vi "PLC to MES monitor - old.vi"(0 "UTP IO Session in":T1, 5 "Sequence Context In":refnum<k7>, 7 "Logged In":bool, 9 "Packaging Performed":bool, 11 "error in":errorcluster) -> (4 "UTP IO Session out":T1, 15 "error out":errorcluster)   [LabVIEW 2023]
uses:
  <vilib>/Noffz/UTP IO/UTP IO Library/Typedefs/Session Handle.ctl
  <vilib>/Noffz/UTP IO/UTP IO Library/UTP IO Pool Session.lvclass
  MES/RequestData.ctl
  5ea416fa-7da9-46cf-b64f-edb3a1b9c4c5.vi
  <vilib>/Noffz/UTP IO/UTP IO Library/methods/poly/plc/Read PLC Variable (Boolean).vi
  <vilib>/Noffz/UTP IO/UTP IO Library/methods/poly/plc/Write PLC Variable (Boolean).vi
  <vilib>/Noffz/UTP IO/UTP IO Library/methods/poly/plc/Write PLC Variable (I16).vi
  <vilib>/addons/TestStand/_TSUtility.llb/TestStand - Get Property Value (Boolean).vi
  <vilib>/addons/TestStand/_TSUtility.llb/TestStand - Get Property Value (String).vi
panel:
  in  "stop":bool
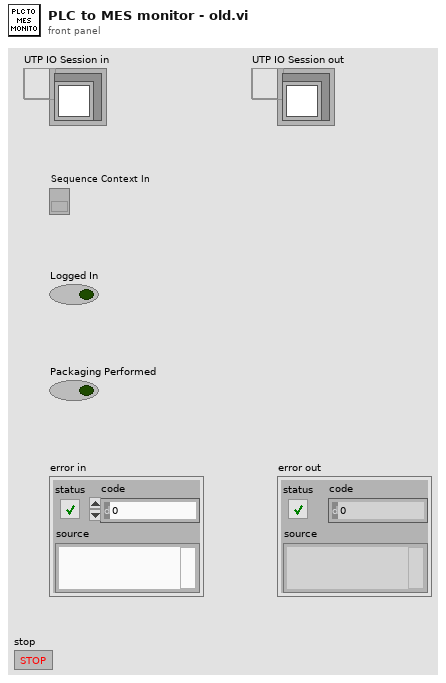
[diagram p1: front panel]
types:
  T1 = typedef "UTP IO Library.lvlib/UTP IO Pool Session.lvclass/Session Handle.ctl" = refnum<data-value>
  T2 = typedef "RequestData.ctl" = cluster{"SOAP":cluster{"HuNo":string, "MaterialCode":string, "Mode":i32, "Operator":string, "PackingInstructions":string, "ProductionVersion":string, "SerialNo":string}, "HU Validation":cluster{"MaterialCode":string, "Operator":string, "SerialNo":string}, "Login":cluster{"EquipmentCode":string, "Mode":i32, "Operator":string}}
  T3 = typedef "TestStand - Status Monitor.ctl" = cluster{"Sequence Context":refnum<k7>, "Execution":refnum<k7>, "Termination Monitor":refnum<k7>}
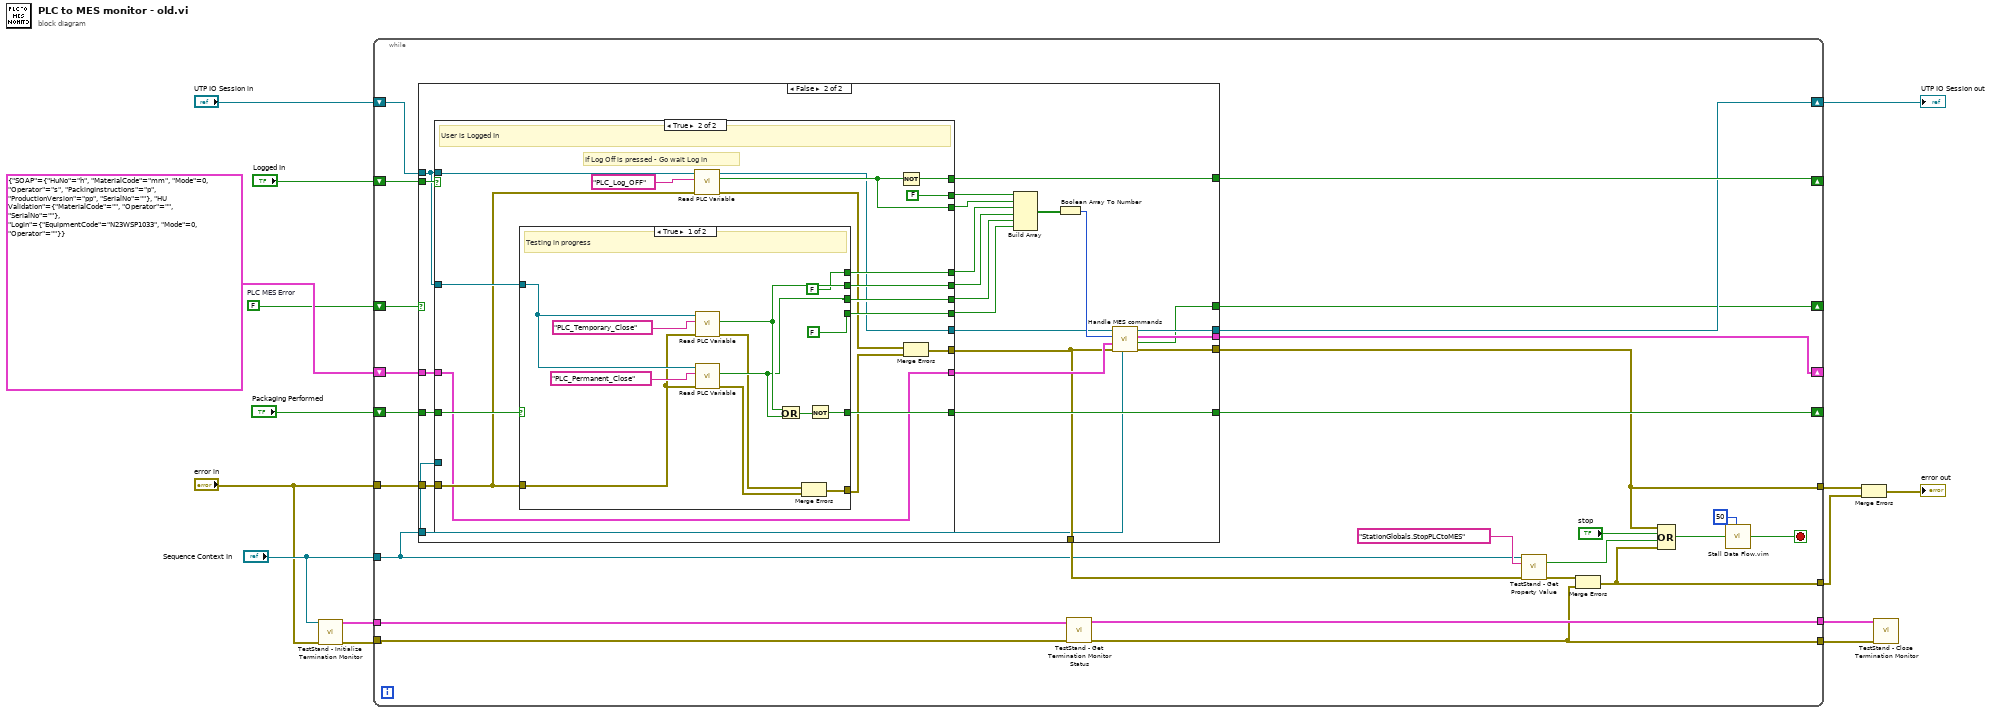
[diagram p0: block diagram]
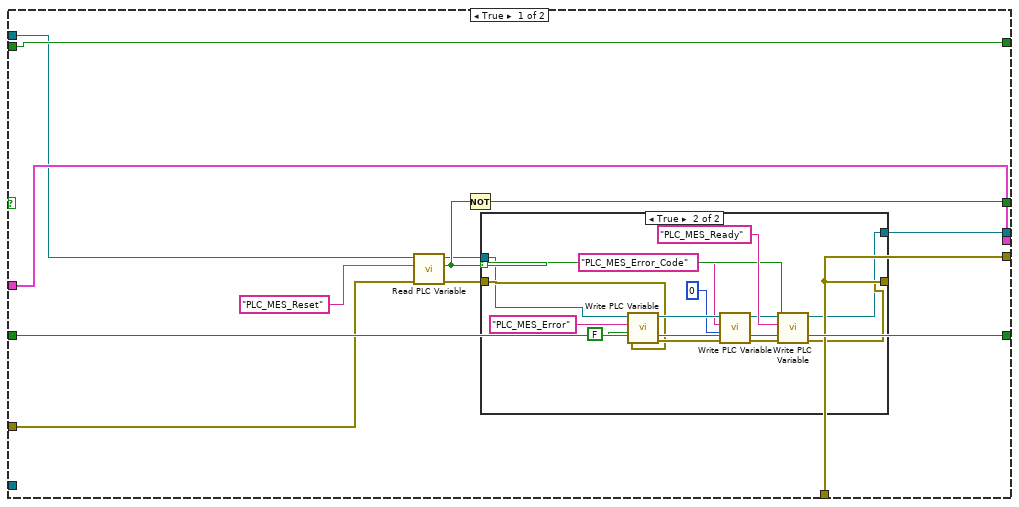
[diagram p2: hidden frame]
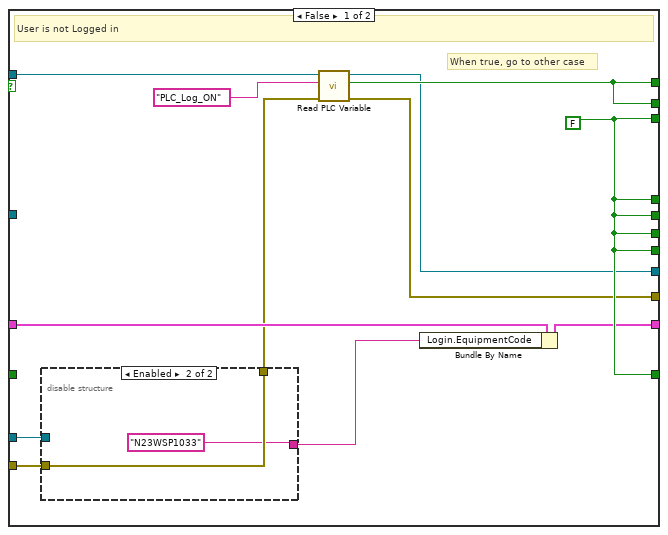
[diagram p4: hidden frame]
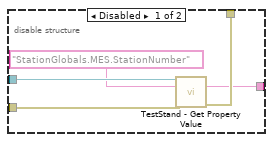
[diagram p5: hidden frame]
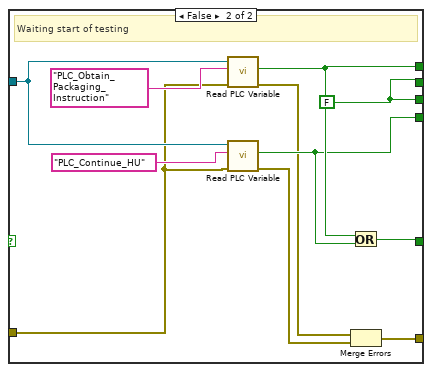
[diagram p6: hidden frame]
diagram:
  w1 = FALSE  # PLC MES Error
  n1 = call <vilib>:"TestStand - Initialize Termination Monitor.vi"("error in (no error)"="error in", "Sequence Context In"="Sequence Context In") -> ("error out"=w11:errorcluster, "Status Monitor Out"=w9:T3)  [unwired: 8 in]
  n2 = while {
    shift-right: [w25] -> w14
    shift-left: "UTP IO Session in" -> [w26]
    shift-right: [w40] -> _
    shift-left: "Logged In" -> [w41]
    shift-right: [w38] -> _
    shift-left: "Packaging Performed" -> [w39]
    tunnel: w11 -> [w37]
    tunnel: [w29] -> w10
    tunnel: w9 -> [w36]
    tunnel: [w35] -> w8
    tunnel: "Sequence Context In" -> [w18]
    tunnel: "error in" -> [w28]
    tunnel: [w20] -> w5
    tunnel: [w27] -> w3
    shift-right: [w23] -> _
    shift-left: T2 {"SOAP"={"HuNo"="h", "MaterialCode"="mm", "Mode"=0, "Operator"="s", "PackingInstructions"="p", "ProductionVersion"="pp", "SerialNo"=""}, "HU Validation"={"MaterialCode"="", "Operator"="", "SerialNo"=""}, "Login"={"EquipmentCode"="N23WSP1033", "Mode"=0, "Operator"=""}} ("RequestData") -> [w24]
    shift-right: [w16] -> _
    shift-left: w1 -> [w17]
    stop <- w22 stop-if-true
    n3 = case shown="False" w17 {
      tunnel: w41 -> [w53 w92]
      tunnel: [w53 w91] -> w40
      tunnel: w39 -> [w51 w87]
      tunnel: [w51 w86] -> w38
      tunnel: w28 -> [w49 w80]
      tunnel: w26 -> [w50 w79]
      tunnel: [w44 w77] -> w25
      tunnel: w24 -> [w52 w75]
      tunnel: [w52 w74] -> w23
      tunnel: [w42 w73] -> w20
      tunnel: [w42 w72] -> w19
      tunnel: w18 -> [_ w71]
      tunnel: [w47 w70] -> w16
      frame True {
        n4 = call-poly <vilib>:"Read PLC Variable.vi"("error in (no error)"=w49, "variable name"="PLC_MES_Reset", "UTP IO Session in"=w50) -> ("error out"=w43:errorcluster, "value"=w46:bool, "UTP IO Session out"=w45:T1)  [unwired: 6 in]
        n5 = Not(x=w46) -> (.not. x?=w47:bool)
        n6 = case shown="True" w46 {
          selector: w46 -> [_ w68]
          tunnel: w45 -> [w55 w60]
          tunnel: [w55 w59] -> w44
          tunnel: w43 -> [w54 w63]
          tunnel: [w54 w61] -> w42
          frame False {
          }
          frame True {
            n7 = call-poly <vilib>:"Write PLC Variable.vi"("error in (no error)"=w63, "value"=FALSE, "variable name"="PLC_MES_Error", "UTP IO Session in"=w60) -> ("error out"=w66:errorcluster, "UTP IO Session out"=w67:T1)  [unwired: 6 in]
            n8 = call-poly <vilib>:"Write PLC Variable.vi"("error in (no error)"=w66, "value"=i16 0, "variable name"="PLC_MES_Error_Code", "UTP IO Session in"=w67) -> ("error out"=w62:errorcluster, "UTP IO Session out"=w56:T1)  [unwired: 6 in]
            n9 = call-poly <vilib>:"Write PLC Variable.vi"("error in (no error)"=w62, "value"=w68, "variable name"="PLC_MES_Ready", "UTP IO Session in"=w56) -> ("error out"=w61:errorcluster, "UTP IO Session out"=w59:T1)  [unwired: 6 in]
          }
        }
      }
      frame False {
        n10 = case shown="True" w92 {
          tunnel: w79 -> [w103 w128]
          tunnel: [w102 w127] -> w91
          tunnel: w79 -> [_ w126]
          tunnel: [w101 w125] -> w88
          tunnel: [w102 FALSE ("value")] -> w89
          tunnel: w87 -> [_ w123]
          tunnel: [w101 w122] -> w85
          tunnel: [w101 w121] -> w84
          tunnel: [w101 w120] -> w83
          tunnel: [w101 w119] -> w86
          tunnel: [w101 w118] -> w82
          tunnel: w80 -> [w96 w117]
          tunnel: [w100 w116] -> w72
          tunnel: [w99 w113] -> w78
          tunnel: [w94 w112] -> w76
          tunnel: w75 -> [w98 w112]
          tunnel: w71 -> [w97 _]
          frame False {
            w101 = FALSE ("value")
            # "When true, go to other case"
            # "User is not Logged in"
            n11 = disable-structure shown="Enabled" {
              disable-tunnel: w97 -> [w109 _]
              disable-tunnel: w96 -> [w108 w111]
              disable-tunnel: [w106 w111] -> w95
              disable-tunnel: [w105 "N23WSP1033" ("Value")] -> w93
              frame Disabled {
                n12 = call-poly <vilib>:"TestStand - Get Property Value.vi"("Sequence Context In"=w109, "Lookup String"="StationGlobals.MES.StationNumber", "error in (no error)"=w108) -> ("Value"=w105:string, "error out"=w106:errorcluster)  [unwired: 10 in, 1 out]
              }
              frame Enabled {
              }
            }
            n13 = call-poly <vilib>:"Read PLC Variable.vi"("error in (no error)"=w95, "variable name"="PLC_Log_ON", "UTP IO Session in"=w103) -> ("error out"=w100:errorcluster, "value"=w102:bool, "UTP IO Session out"=w99:T1)  [unwired: 6 in]
            n14 = Bundle By Name(cluster=w98, "Login.EquipmentCode"=w93) -> (w94:T2)
          }
          frame True {
            # "If Log Off is pressed - Go wait Log in"
            # "User is Logged In"
            n15 = case shown="True" w123 {
              tunnel: w126 -> [w140 w150]
              tunnel: [FALSE ("value") w148] -> w122
              tunnel: [w139 w152] -> w121
              tunnel: [w138 w152] -> w120
              tunnel: [w136 w149] -> w119
              tunnel: [FALSE ("value") w147] -> w118
              tunnel: w117 -> [w133 w145]
              tunnel: [w130 w146] -> w115
              frame True {
                # "Testing in progress"
                n16 = call-poly <vilib>:"Read PLC Variable.vi"("error in (no error)"=w133, "variable name"="PLC_Temporary_Close", "UTP IO Session in"=w140) -> ("error out"=w132:errorcluster, "value"=w139:bool)  [unwired: 6 in, 1 out]
                n17 = call-poly <vilib>:"Read PLC Variable.vi"("error in (no error)"=w133, "variable name"="PLC_Permanent_Close", "UTP IO Session in"=w140) -> ("error out"=w131:errorcluster, "value"=w138:bool)  [unwired: 6 in, 1 out]
                n18 = Or(x=w139, y=w138) -> (x .or. y?=w137:bool)
                n19 = Merge Errors(w132, w131) -> (w130:errorcluster)
                n20 = Not(x=w137) -> (.not. x?=w136:bool)
              }
              frame False {
                w152 = FALSE ("value")
                # "Waiting start of testing"
                n21 = call-poly <vilib>:"Read PLC Variable.vi"("error in (no error)"=w145, "variable name"="PLC_Obtain_Packaging_Instruction", "UTP IO Session in"=w150) -> ("error out"=w144:errorcluster, "value"=w148:bool)  [unwired: 6 in, 1 out]
                n22 = call-poly <vilib>:"Read PLC Variable.vi"("error in (no error)"=w145, "variable name"="PLC_Continue_HU", "UTP IO Session in"=w150) -> ("error out"=w143:errorcluster, "value"=w147:bool)  [unwired: 6 in, 1 out]
                n23 = Or(x=w148, y=w147) -> (x .or. y?=w149:bool)
                n24 = Merge Errors(w144, w143) -> (w146:errorcluster)
              }
            }
            n25 = call-poly <vilib>:"Read PLC Variable.vi"("error in (no error)"=w117, "variable name"="PLC_Log_OFF", "UTP IO Session in"=w128) -> ("error out"=w114:errorcluster, "value"=w125:bool, "UTP IO Session out"=w113:T1)  [unwired: 6 in]
            n26 = Not(x=w125) -> (.not. x?=w127:bool)
            n27 = Merge Errors(w114, w115) -> (w116:errorcluster)
          }
        }
        n28 = Build Array(w89, w88, w85, w84, w83, w82) -> (w90:bool[])
        n29 = Boolean Array To Number(Boolean array=w90) -> (number=w81:u32)
        n30 = call "Handle MES commands.vi"("Sequence Context In"=w71, "error in (no error)"=w72, "RequestData in"=w76, "Request"=w81, "Data Value Reference in"=w78) -> ("error out"=w73:errorcluster, "PLC MES Error"=w70:bool, "RequestData out"=w74:T2, "Data Value Reference out"=w77:T1)  [unwired: 3 in]
      }
    }
    n31 = call <vilib>:"TestStand - Get Termination Monitor Status.vi"("error in (no error)"=w37, "Status Monitor In"=w36) -> ("error out"=w29:errorcluster, "Status Monitor Out"=w35:T3)  [unwired: 7 in, 1 out]
    n32 = call-poly <vilib>:"TestStand - Get Property Value.vi"("Sequence Context In"=w18, "Lookup String"="StationGlobals.StopPLCtoMES", "error in (no error)"=w19) -> ("Value"=w31:bool, "error out"=w30:errorcluster)  [unwired: 10 in, 1 out]
    n33 = Merge Errors(w30, w29) -> (w27:errorcluster)
    n34 = Compound Arithmetic op=OR(w20, "stop", w31, w27) -> (w32:bool)
    n35 = call "Stall Data Flow.vim"("value in"=w32, "milliseconds to wait"=u32 50) -> ("value out"=w22:bool)  [unwired: 1 out]
  }
  "UTP IO Session out" <- w14
  n36 = Merge Errors(w5, w3) -> (→"error out":errorcluster)
  n37 = call <vilib>:"TestStand - Close Termination Monitor.vi"("error in (no error)"=w10, "Status Monitor In"=w8) -> ()  [unwired: 9 in, 1 out]
